vi "SetStop.vi"(8 "error in":errorcluster, 11 "VISA resource name":refnum<visa-resource-name>) -> (0 "error out":errorcluster, 3 "VISA resource name out":refnum<visa-resource-name>)   [LabVIEW 2023, in "Thermotron 8800.lvlib"]
doc: "STOP\n\nCommand name: Stop controller\nCommand type: Control\nDescription: Places the 8800 in stop mode.\nSyntax: STOP\nData type: No data\nQuery example: STOP\n8800 response: The 8800 goes into stop mode"
uses:
  Thermotron 8800.lvlib
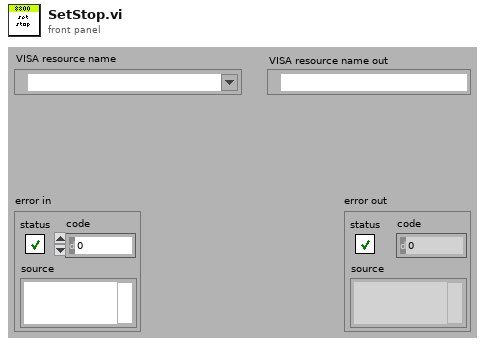
[diagram p1: front panel]
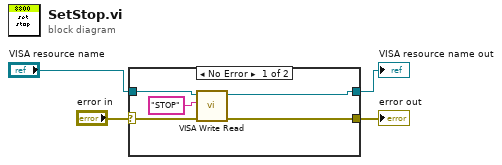
[diagram p0: block diagram]
diagram:
  n1 = case shown="No Error" "error in" {
    selector: "error in" -> [w5 w10]
    tunnel: "VISA resource name" -> [w8 w11]
    tunnel: [w7 w11] -> w3
    tunnel: [w6 w10] -> w2
    frame No Error {
      n2 = call "VISA Write Read.vi"("error in (no error)"=w5, "8800 Command"="STOP", "VISA Refnum in"=w8) -> ("error out"=w6:errorcluster, "VISA Refnum out"=w7:refnum<visa-resource-name>)  [unwired: 6 in, 1 out]
    }
    frame Error {
      # "execute no code if incoming error"
    }
  }
  "VISA resource name out" <- w3
  "error out" <- w2
